vi "采集参数设置.vi"() -> (3 "Cancelled?":bool)   [LabVIEW 2020]
uses:
  global/SettingVariable.vi
  <vilib>/Utility/config.llb/Write Key (Double).vi
  <vilib>/Utility/config.llb/Write Key (Boolean).vi
  <vilib>/Utility/config.llb/Write Key (String).vi
  <vilib>/Utility/config.llb/Write Key (U32).vi
  <vilib>/Utility/config.llb/Write Key (I32).vi
  <vilib>/Utility/config.llb/NI_LVConfig.lvlib
panel:
  in  "电压范围8":cluster{"Numeric":i32, "Numeric":i32}(slide)={"Numeric"=5, "Numeric"=1} scale=-10.0..10.0
  in  "电压范围7":cluster{"Numeric":i32, "Numeric":i32}(slide)={"Numeric"=5, "Numeric"=1} scale=-10.0..10.0
  in  "电压范围6":cluster{"Numeric":i32, "Numeric":i32}(slide)={"Numeric"=5, "Numeric"=1} scale=-10.0..10.0
  in  "电压范围5":cluster{"Numeric":i32, "Numeric":i32}(slide)={"Numeric"=5, "Numeric"=1} scale=-10.0..10.0
  in  "电压范围4":cluster{"Numeric":i32, "Numeric":i32}(slide)={"Numeric"=5, "Numeric"=1} scale=-10.0..10.0
  in  "电压范围3":cluster{"Numeric":i32, "Numeric":i32}(slide)={"Numeric"=5, "Numeric"=1} scale=-10.0..10.0
  in  "电压范围2":cluster{"Numeric":i32, "Numeric":i32}(slide)={"Numeric"=5, "Numeric"=1} scale=-10.0..10.0
  in  "电压范围1":cluster{"Numeric":i32, "Numeric":i32}(slide)={"Numeric"=5, "Numeric"=1} scale=-10.0..10.0
  in  "物理量8下限":sgl format="%#.4g"
  in  "物理量8上限":sgl format="%#.4g"
  in  "物理量7下限":sgl format="%#.4g"
  in  "物理量7上限":sgl format="%#.4g"
  in  "物理量6下限":sgl format="%#.4g"
  in  "物理量6上限":sgl format="%#.4g"
  in  "物理量5下限":sgl format="%#.4g"
  in  "物理量5上限":sgl format="%#.4g"
  in  "物理量4下限":sgl format="%#.4g"
  in  "物理量4上限":sgl format="%#.4g"
  in  "物理量3下限":sgl format="%#.4g"
  in  "物理量3上限":sgl format="%#.4g"
  in  "物理量2下限":sgl format="%#.4g"
  in  "物理量2上限":sgl format="%#.4g"
  in  "物理量1下限":sgl format="%#.4g"
  in  "物理量1上限":sgl format="%#.4g"
  in  "电压标尺8":u16(ring) items=["计数通量LOG", "电压通量", "电流通量LOG", "棒位", "温度", "P2参数", "硼浓度"]
  in  "电压标尺7":u16(ring) items=["计数通量LOG", "电压通量", "电流通量LOG", "棒位", "温度", "P2参数", "硼浓度"]
  in  "电压标尺6":u16(ring) items=["计数通量LOG", "电压通量", "电流通量LOG", "棒位", "温度", "P2参数", "硼浓度"]
  in  "电压标尺5":u16(ring) items=["计数通量LOG", "电压通量", "电流通量LOG", "棒位", "温度", "P2参数", "硼浓度"]
  in  "电压标尺4":u16(ring) items=["计数通量LOG", "电压通量", "电流通量LOG", "棒位", "温度", "P2参数", "硼浓度"]
  in  "电压标尺3":u16(ring) items=["计数通量LOG", "电压通量", "电流通量LOG", "棒位", "温度", "P2参数", "硼浓度"]
  in  "电压标尺2":u16(ring) items=["计数通量LOG", "电压通量", "电流通量LOG", "棒位", "温度", "P2参数", "硼浓度"]
  in  "电压标尺1":u16(ring) items=["计数通量LOG", "电压通量", "电流通量LOG", "棒位", "温度", "P2参数", "硼浓度"]
  in  "电流输入名称2":string
  in  "电流输入名称1":string
  in  "电压输入名称8":string
  in  "电压输入名称7":string
  in  "电压输入名称6":string
  in  "电压输入名称5":string
  in  "电压输入名称4":string
  in  "电压输入名称3":string
  in  "电压输入名称2":string
  in  "电压输入名称1":string
  in  "电流输入2":bool
  in  "电流输入1":bool
  in  "电压输入8":bool
  in  "电压输入7":bool
  in  "电压输入6":bool
  in  "电压输入5":bool
  in  "电压输入4":bool
  in  "电压输入3":bool
  in  "电压输入2":bool
  in  "电压输入1":bool
  in  "取消":bool caption="Cancel Button"
  in  "确定":bool
  in  "采集时间间隔":sgl(knob)=0.5 caption="采集时间间隔(s)：" min=0.5 max=2 step=0.5 scale=0.5..2.0 scale format="%#.1f"
  # "仪器通讯"
  # "电压输入通道"
  # "电流输入通道"
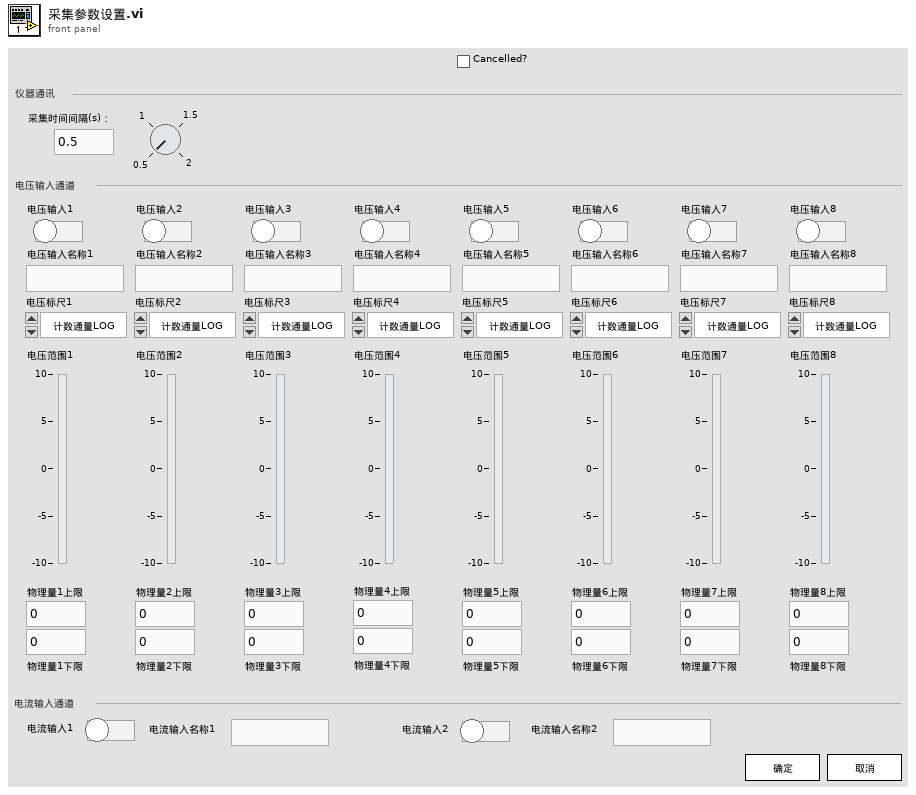
[diagram p1: front panel]
types:
  T1 = cluster{"switch":bool, "name":string, "voltage upper":i32, "voltage lower":i32, "physics upper":dbl, "physics lower":dbl, "scale":u16}[]
  T2 = typedef "NI_LVConfig.lvlib/Config Data RefNum.ctl" = refnum<k1>
  T3 = cluster{"switch":bool, "name":string, "voltage upper":i32, "voltage lower":i32, "physics upper":dbl, "physics lower":dbl, "scale":u16}
  T4 = enum32{"Bad", "Idle", "Run top level", "Running"}
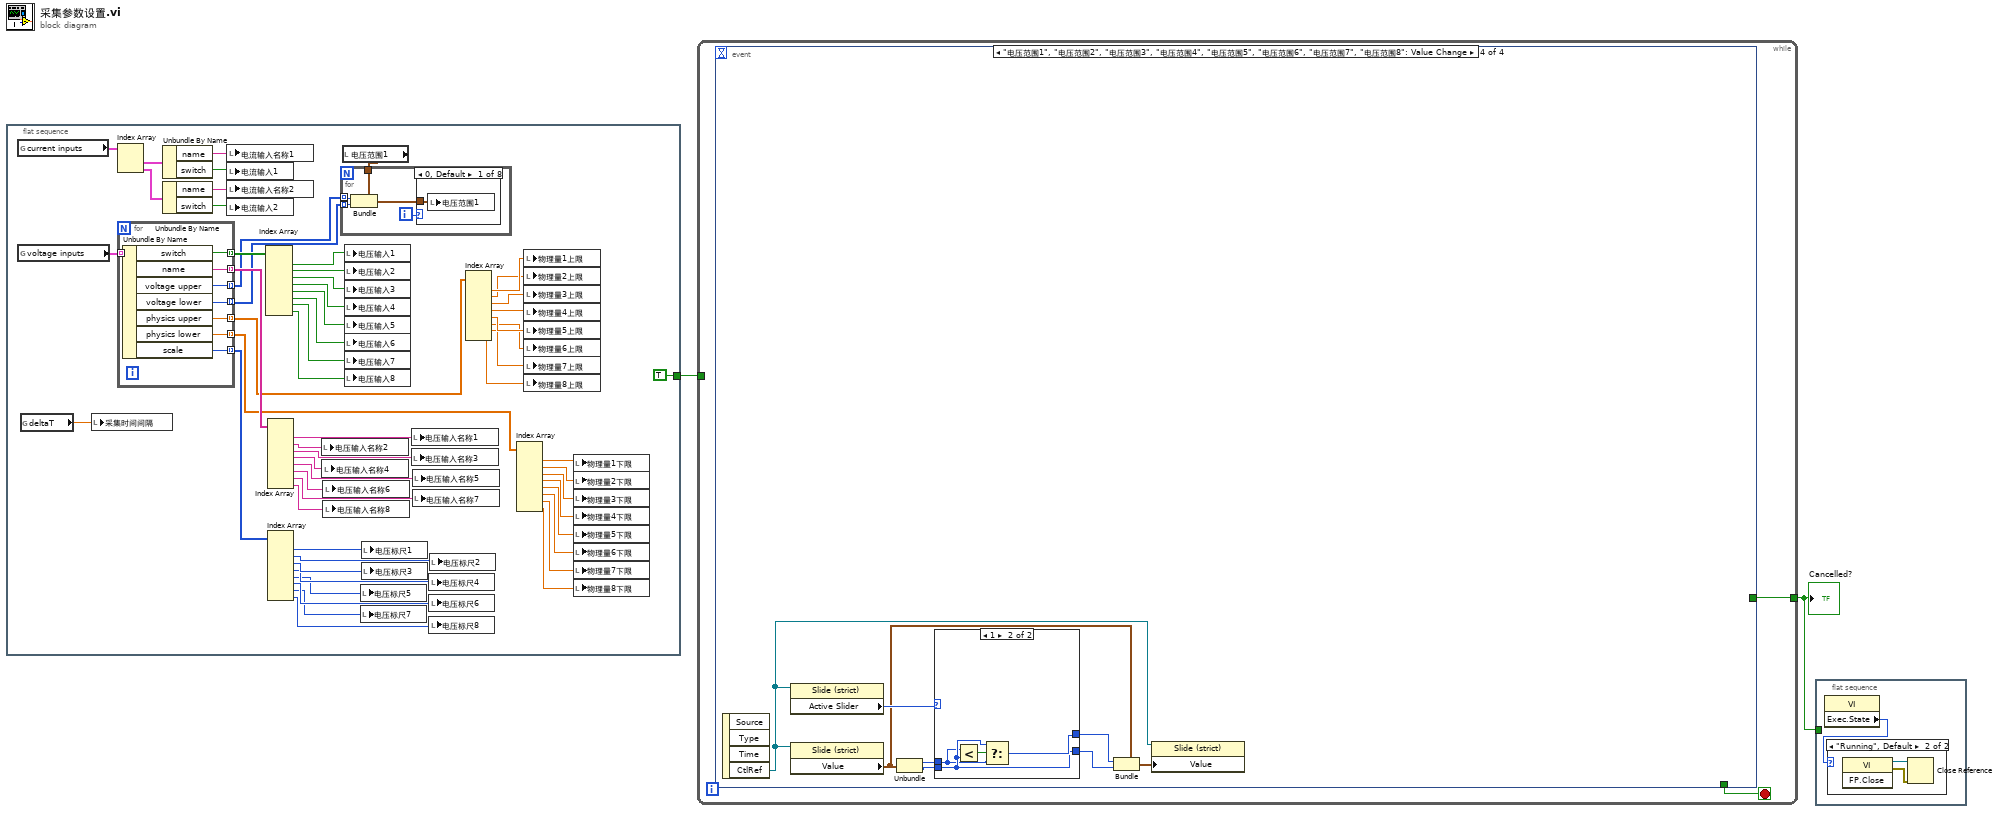
[diagram p0: block diagram]
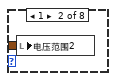
[diagram p3: hidden frame]
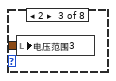
[diagram p4: hidden frame]
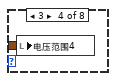
[diagram p5: hidden frame]
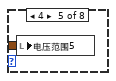
[diagram p6: hidden frame]
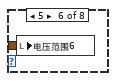
[diagram p7: hidden frame]
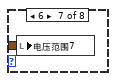
[diagram p8: hidden frame]
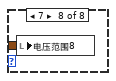
[diagram p9: hidden frame]
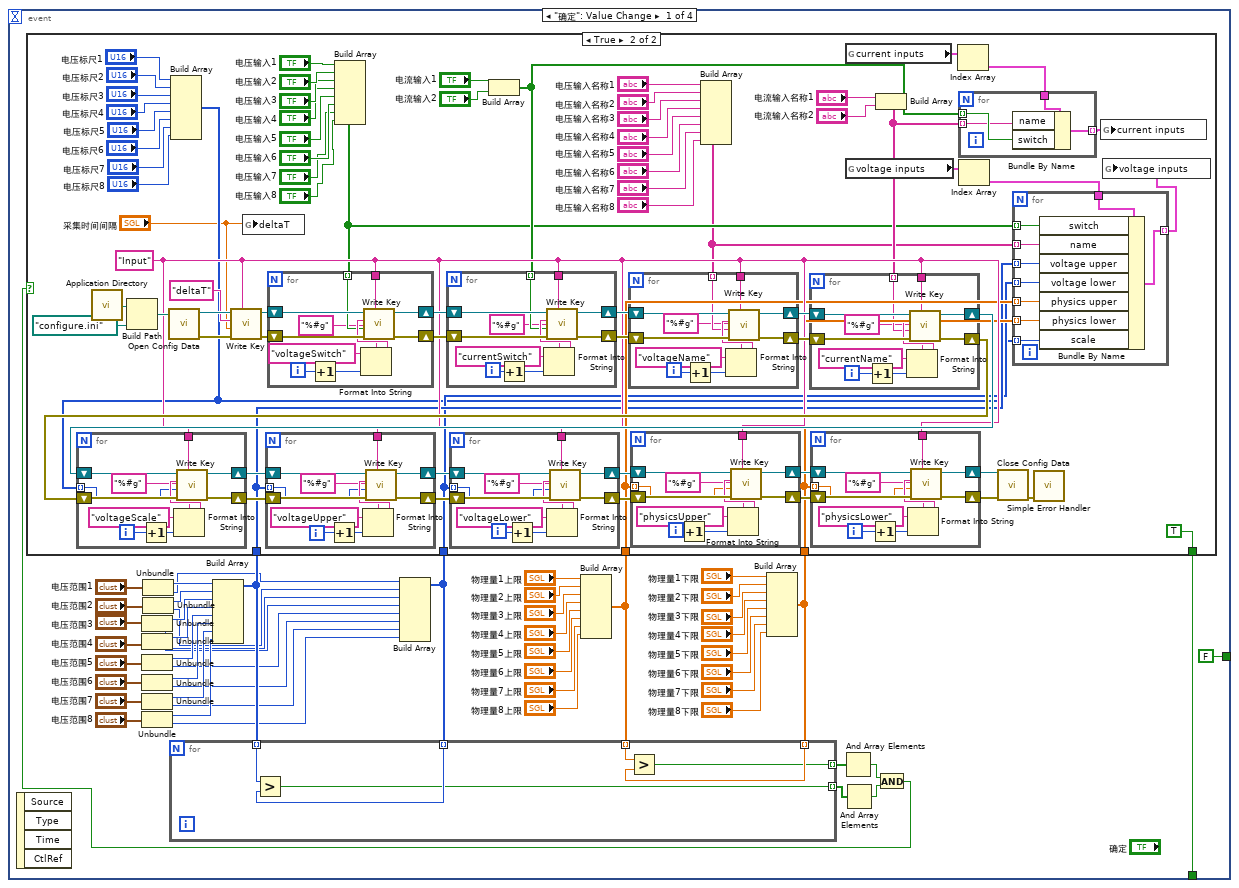
[diagram p10: hidden frame]
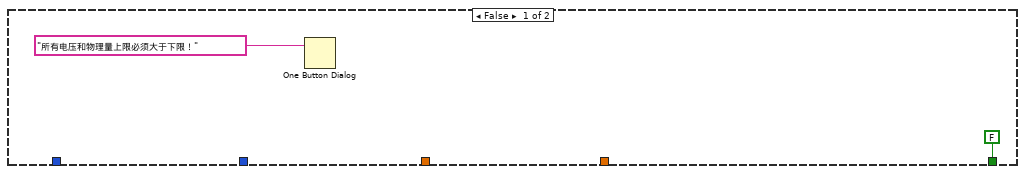
[diagram p11: hidden frame]
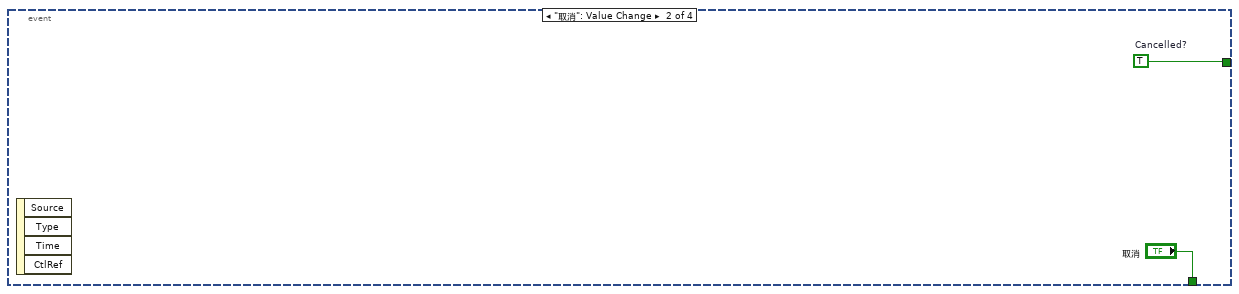
[diagram p12: hidden frame]
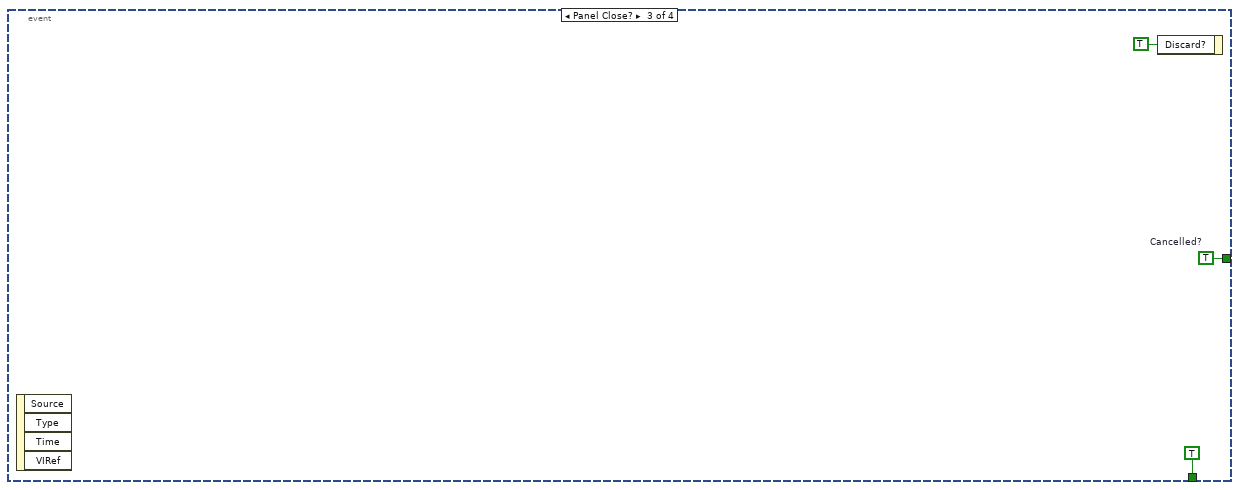
[diagram p13: hidden frame]
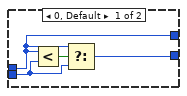
[diagram p14: hidden frame]
diagram:
  n1 = flat-sequence {
    tunnel: [TRUE] -> w2
    frame #0 {
      n2 = global read "SettingVariable.vi" "current inputs"() -> (w59:cluster{"name":string, "switch":bool}[])
      n3 = global read "SettingVariable.vi" "voltage inputs"() -> (w52:T1)
      n4 = global read "SettingVariable.vi" "deltaT"() -> (w60:dbl)
      n5 = local write "采集时间间隔"(w60) -> ()
      n6 = Index Array(array=w59) -> (element #1=w58:cluster{"name":string, "switch":bool}, element #2=w57:cluster{"name":string, "switch":bool})  [unwired: 2 in]
      n7 = for {
        tunnel: w52 -> [w81] mode=indexing
        tunnel: [w80] -> w51 mode=indexing
        tunnel: [w79] -> w41 mode=indexing
        tunnel: [w78] -> w3 mode=indexing
        tunnel: [w77] -> w4 mode=indexing
        tunnel: [w76] -> w23 mode=indexing
        tunnel: [w75] -> w22 mode=indexing
        tunnel: [w74] -> w32 mode=indexing
        n8 = Unbundle By Name(w81) -> ("switch"=w80:bool, "name"=w79:string, "voltage upper"=w78:i32, "voltage lower"=w77:i32, "physics upper"=w76:dbl, "physics lower"=w75:dbl, "scale"=w74:u16)
      }
      n9 = Unbundle By Name(w58) -> ("name"=w56:string, "switch"=w54:bool)
      n10 = Unbundle By Name(w57) -> ("name"=w55:string, "switch"=w53:bool)
      n11 = local write "电流输入名称1"(w56) -> ()
      n12 = local write "电流输入1"(w54) -> ()
      n13 = local write "电流输入名称2"(w55) -> ()
      n14 = local write "电流输入2"(w53) -> ()
      n15 = Index Array(array=w51) -> (element #1=w50:bool, element #2=w49:bool, element #3=w48:bool, element #4=w47:bool, element #5=w46:bool, element #6=w45:bool, element #7=w44:bool, element #8=w43:bool)  [unwired: 8 in]
      n16 = Index Array(array=w41) -> (element #1=w42:string, element #2=w40:string, element #3=w39:string, element #4=w38:string, element #5=w37:string, element #6=w36:string, element #7=w35:string, element #8=w34:string)  [unwired: 8 in]
      n17 = Index Array(array=w32) -> (element #1=w33:u16, element #2=w31:u16, element #3=w30:u16, element #4=w29:u16, element #5=w28:u16, element #6=w27:u16, element #7=w26:u16, element #8=w25:u16)  [unwired: 8 in]
      n18 = local write "电压输入名称2"(w40) -> ()
      n19 = local write "电压输入名称4"(w38) -> ()
      n20 = local write "电压输入名称6"(w36) -> ()
      n21 = local write "电压输入名称8"(w34) -> ()
      n22 = local read "电压范围1"() -> (w5:cluster{"Numeric":i32, "Numeric":i32})
      n23 = for {
        tunnel: w5 -> [w63]
        tunnel: w4 -> [w62] mode=indexing
        tunnel: w3 -> [w61] mode=indexing
        i -> [w64]
        n24 = Bundle(cluster=w63, "Numeric"=w61, "Numeric"=w62) -> (w65:cluster{"Numeric":i32, "Numeric":i32})
        n25 = case shown="0, Default" w64 {
          tunnel: w65 -> [w66 w67 w68 w69 w70 w71 w72 w73]
          frame 0, Default {
            n26 = local write "电压范围1"(w66) -> ()
          }
          frame 1 {
            n27 = local write "电压范围2"(w67) -> ()
          }
          frame 2 {
            n28 = local write "电压范围3"(w68) -> ()
          }
          frame 3 {
            n29 = local write "电压范围4"(w69) -> ()
          }
          frame 4 {
            n30 = local write "电压范围5"(w70) -> ()
          }
          frame 5 {
            n31 = local write "电压范围6"(w71) -> ()
          }
          frame 6 {
            n32 = local write "电压范围7"(w72) -> ()
          }
          frame 7 {
            n33 = local write "电压范围8"(w73) -> ()
          }
        }
      }
      n34 = local write "电压输入1"(w50) -> ()
      n35 = local write "电压输入2"(w49) -> ()
      n36 = local write "电压输入3"(w48) -> ()
      n37 = local write "电压输入4"(w47) -> ()
      n38 = local write "电压输入5"(w46) -> ()
      n39 = local write "电压输入6"(w45) -> ()
      n40 = local write "电压输入7"(w44) -> ()
      n41 = local write "电压输入8"(w43) -> ()
      n42 = local write "电压标尺5"(w28) -> ()
      n43 = local write "电压标尺7"(w26) -> ()
      n44 = local write "电压标尺1"(w33) -> ()
      n45 = local write "电压标尺3"(w30) -> ()
      n46 = local write "电压输入名称1"(w42) -> ()
      n47 = local write "电压输入名称3"(w39) -> ()
      n48 = local write "电压输入名称5"(w37) -> ()
      n49 = local write "电压输入名称7"(w35) -> ()
      n50 = local write "电压标尺4"(w29) -> ()
      n51 = local write "电压标尺6"(w27) -> ()
      n52 = local write "电压标尺8"(w25) -> ()
      n53 = local write "电压标尺2"(w31) -> ()
      n54 = Index Array(array=w23) -> (element #1=w24:dbl, element #2=w21:dbl, element #3=w20:dbl, element #4=w19:dbl, element #5=w18:dbl, element #6=w17:dbl, element #7=w16:dbl, element #8=w15:dbl)  [unwired: 8 in]
      n55 = Index Array(array=w22) -> (element #1=w14:dbl, element #2=w13:dbl, element #3=w12:dbl, element #4=w11:dbl, element #5=w10:dbl, element #6=w9:dbl, element #7=w8:dbl, element #8=w7:dbl)  [unwired: 8 in]
      n56 = local write "物理量1上限"(w24) -> ()
      n57 = local write "物理量2上限"(w21) -> ()
      n58 = local write "物理量3上限"(w20) -> ()
      n59 = local write "物理量4上限"(w19) -> ()
      n60 = local write "物理量5上限"(w18) -> ()
      n61 = local write "物理量6上限"(w17) -> ()
      n62 = local write "物理量7上限"(w16) -> ()
      n63 = local write "物理量8上限"(w15) -> ()
      n64 = local write "物理量1下限"(w14) -> ()
      n65 = local write "物理量2下限"(w13) -> ()
      n66 = local write "物理量3下限"(w12) -> ()
      n67 = local write "物理量4下限"(w11) -> ()
      n68 = local write "物理量5下限"(w10) -> ()
      n69 = local write "物理量6下限"(w9) -> ()
      n70 = local write "物理量7下限"(w8) -> ()
      n71 = local write "物理量8下限"(w7) -> ()
    }
  }
  n72 = while {
    tunnel: w2 -> [_]
    tunnel: [w82] -> w1
    stop <- w83 stop-if-true
    n73 = event shown="[3] \"电压范围1\", \"电压范围2\", \"电压范围3\", \"电压范围4\", \"电压范围5\", \"电压范围6\", \"电压范围7\", \"电压范围8\": Value Change" {
      selector: _ -> [_ _ _ _]
      dyn-events: _ -> [_ _ _ _]
      timeout: _ -> [_ _ _ _]
      tunnel: [w112 "取消" TRUE _] -> w83
      tunnel: [FALSE ("Cancelled?") w328 w330 _] -> w82
      event "确定": Value Change {
        n74 = event-data() -> ()  [unwired: 1 in, 4 out]
        n75 = Unbundle("电压范围3") -> ("Numeric"=w97:i32, "Numeric"=w89:i32)
        n76 = Unbundle("电压范围4") -> ("Numeric"=w96:i32, "Numeric"=w88:i32)
        n77 = Unbundle("电压范围5") -> ("Numeric"=w94:i32, "Numeric"=w87:i32)
        n78 = Unbundle("电压范围6") -> ("Numeric"=w93:i32, "Numeric"=w86:i32)
        n79 = Unbundle("电压范围7") -> ("Numeric"=w92:i32, "Numeric"=w85:i32)
        n80 = Unbundle("电压范围8") -> ("Numeric"=w91:i32, "Numeric"=w84:i32)
        n81 = Unbundle("电压范围1") -> ("Numeric"=w99:i32, "Numeric"=w95:i32)
        n82 = Unbundle("电压范围2") -> ("Numeric"=w98:i32, "Numeric"=w90:i32)
        n83 = Build Array(w99, w98, w97, w96, w94, w93, w92, w91) -> (w121:i32[])
        n84 = Build Array(w95, w90, w89, w88, w87, w86, w85, w84) -> (w120:i32[])
        n85 = Build Array("物理量1上限", "物理量2上限", "物理量3上限", "物理量4上限", "物理量5上限", "物理量6上限", "物理量7上限", "物理量8上限") -> (w119:sgl[])
        n86 = Build Array("物理量1下限", "物理量2下限", "物理量3下限", "物理量4下限", "物理量5下限", "物理量6下限", "物理量7下限", "物理量8下限") -> (w118:sgl[])
        n87 = for {
          tunnel: w121 -> [w327] mode=indexing
          tunnel: w120 -> [w326] mode=indexing
          tunnel: w119 -> [w325] mode=indexing
          tunnel: w118 -> [w324] mode=indexing
          tunnel: [w323] -> w117 mode=indexing
          tunnel: [w322] -> w116 mode=indexing
          n88 = Greater?(x=w327, y=w326) -> (0:w322:bool)
          n89 = Greater?(x=w325, y=w324) -> (0:w323:bool)
        }
        n90 = And Array Elements(Boolean array=w117) -> (logical AND=w114:bool)
        n91 = And Array Elements(Boolean array=w116) -> (logical AND=w115:bool)
        n92 = And(x=w114, y=w115) -> (x .and. y?=w113:bool)
        n93 = case shown="True" w113 {
          tunnel: w121 -> [_ w140]
          tunnel: w120 -> [_ w139]
          tunnel: w119 -> [_ w142]
          tunnel: w118 -> [_ w141]
          tunnel: [FALSE TRUE] -> w112
          frame False {
            n94 = One Button Dialog(message="所有电压和物理量上限必须大于下限！") -> ()  [unwired: 1 in, 1 out]
          }
          frame True {
            w156 = "Input" ("section")
            n95 = call <vilib>:"Application Directory.vi"() -> ("Application Directory"=w180:path)
            n96 = Build Path(base path=w180, name or relative path=path "configure.ini") -> (appended path=w178:path)
            n97 = call <vilib>:"Open Config Data.vi"("configuration file path"=w178) -> ("error out"=w176:errorcluster, "refnum"=w177:T2)  [unwired: 2 in, 7 out]
            n98 = Build Array("电压标尺1", "电压标尺2", "电压标尺3", "电压标尺4", "电压标尺5", "电压标尺6", "电压标尺7", "电压标尺8") -> (w138:u16[])
            n99 = call-poly <vilib>:"Write Key.vi"("section"=w156, "error in (no error)"=w176, "value"="采集时间间隔", "key"="deltaT", "refnum"=w177) -> ("error out"=w173:errorcluster, "refnum out"=w174:T2)  [unwired: 4 in, 1 out]
            n100 = global write "SettingVariable.vi" "deltaT"("采集时间间隔") -> ()
            n101 = Build Array("电压输入1", "电压输入2", "电压输入3", "电压输入4", "电压输入5", "电压输入6", "电压输入7", "电压输入8") -> (w144:bool[])
            n102 = for {
              tunnel: w144 -> [w316] mode=indexing
              shift-right: [w315] -> w172
              shift-left: w174 -> [w321]
              shift-right: [w314] -> w171
              shift-left: w173 -> [w320]
              tunnel: w156 -> [w312]
              i -> [w319]
              n103 = Increment(x=w319) -> (x+1=w311:i32)
              n104 = Format Into String(format string="%#g" ("section"), initial string="voltageSwitch", w311) -> (resulting string=w317:string)  [unwired: 1 in, 1 out]
              n105 = call-poly <vilib>:"Write Key.vi"("section"=w312, "error in (no error)"=w320, "value"=w316, "key"=w317, "refnum"=w321) -> ("error out"=w314:errorcluster, "refnum out"=w315:T2)  [unwired: 4 in, 1 out]
            }
            n106 = Build Array("电流输入1", "电流输入2") -> (w151:bool[])
            n107 = for {
              tunnel: w151 -> [w305] mode=indexing
              shift-right: [w303] -> w169
              shift-left: w172 -> [w310]
              shift-right: [w304] -> w170
              shift-left: w171 -> [w309]
              tunnel: w156 -> [w301]
              i -> [w308]
              n108 = Increment(x=w308) -> (x+1=w300:i32)
              n109 = Format Into String(format string="%#g" ("section"), initial string="currentSwitch", w300) -> (resulting string=w306:string)  [unwired: 1 in, 1 out]
              n110 = call-poly <vilib>:"Write Key.vi"("section"=w301, "error in (no error)"=w309, "value"=w305, "key"=w306, "refnum"=w310) -> ("error out"=w304:errorcluster, "refnum out"=w303:T2)  [unwired: 4 in, 1 out]
            }
            n111 = Build Array("电压输入名称1", "电压输入名称2", "电压输入名称3", "电压输入名称4", "电压输入名称5", "电压输入名称6", "电压输入名称7", "电压输入名称8") -> (w143:string[])
            n112 = for {
              tunnel: w143 -> [w294] mode=indexing
              tunnel: w156 -> [w292]
              shift-right: [w291] -> w168
              shift-left: w169 -> [w299]
              shift-right: [w290] -> w167
              shift-left: w170 -> [w298]
              i -> [w297]
              n113 = Increment(x=w297) -> (x+1=w289:i32)
              n114 = Format Into String(format string="%#g" ("section"), initial string="voltageName", w289) -> (resulting string=w295:string)  [unwired: 1 in, 1 out]
              n115 = call-poly <vilib>:"Write Key.vi"("section"=w292, "error in (no error)"=w298, "value"=w294, "key"=w295, "refnum"=w299) -> ("error out"=w290:errorcluster, "refnum out"=w291:T2)  [unwired: 4 in, 1 out]
            }
            n116 = global read "SettingVariable.vi" "current inputs"() -> (w150:cluster{"name":string, "switch":bool}[])
            n117 = global read "SettingVariable.vi" "voltage inputs"() -> (w147:T1)
            n118 = Build Array("电流输入名称1", "电流输入名称2") -> (w152:string[])
            n119 = for {
              tunnel: w152 -> [w283] mode=indexing
              tunnel: w156 -> [w281]
              shift-right: [w280] -> w158
              shift-left: w168 -> [w288]
              shift-right: [w279] -> w157
              shift-left: w167 -> [w287]
              i -> [w286]
              n120 = Increment(x=w286) -> (x+1=w278:i32)
              n121 = Format Into String(format string="%#g" ("section"), initial string="currentName", w278) -> (resulting string=w284:string)  [unwired: 1 in, 1 out]
              n122 = call-poly <vilib>:"Write Key.vi"("section"=w281, "error in (no error)"=w287, "value"=w283, "key"=w284, "refnum"=w288) -> ("error out"=w279:errorcluster, "refnum out"=w280:T2)  [unwired: 4 in, 1 out]
            }
            n123 = for {
              tunnel: w156 -> [w228]
              shift-right: [w227] -> w160
              shift-left: w158 -> [w233]
              shift-right: [w226] -> w159
              shift-left: w157 -> [w232]
              tunnel: w138 -> [w225] mode=indexing
              i -> [w224]
              n124 = Increment(x=w224) -> (x+1=w223:i32)
              n125 = Format Into String(format string="%#g" ("section"), initial string="voltageScale", w223) -> (resulting string=w230:string)  [unwired: 1 in, 1 out]
              n126 = call-poly <vilib>:"Write Key.vi"("section"=w228, "error in (no error)"=w232, "value"=w225, "key"=w230, "refnum"=w233) -> ("error out"=w226:errorcluster, "refnum out"=w227:T2)  [unwired: 4 in, 1 out]
            }
            n127 = for {
              tunnel: w156 -> [w271]
              shift-right: [w270] -> w166
              shift-left: w160 -> [w277]
              shift-right: [w269] -> w165
              shift-left: w159 -> [w276]
              tunnel: w140 -> [w268] mode=indexing
              i -> [w275]
              n128 = Increment(x=w275) -> (x+1=w267:i32)
              n129 = Format Into String(format string="%#g" ("section"), initial string="voltageUpper", w267) -> (resulting string=w273:string)  [unwired: 1 in, 1 out]
              n130 = call-poly <vilib>:"Write Key.vi"("section"=w271, "error in (no error)"=w276, "value"=w268, "key"=w273, "refnum"=w277) -> ("error out"=w269:errorcluster, "refnum out"=w270:T2)  [unwired: 4 in, 1 out]
            }
            n131 = for {
              tunnel: w156 -> [w260]
              shift-right: [w259] -> w164
              shift-left: w166 -> [w266]
              shift-right: [w258] -> w163
              shift-left: w165 -> [w265]
              tunnel: w139 -> [w257] mode=indexing
              i -> [w264]
              n132 = Increment(x=w264) -> (x+1=w256:i32)
              n133 = Format Into String(format string="%#g" ("section"), initial string="voltageLower", w256) -> (resulting string=w262:string)  [unwired: 1 in, 1 out]
              n134 = call-poly <vilib>:"Write Key.vi"("section"=w260, "error in (no error)"=w265, "value"=w257, "key"=w262, "refnum"=w266) -> ("error out"=w258:errorcluster, "refnum out"=w259:T2)  [unwired: 4 in, 1 out]
            }
            n135 = for {
              tunnel: w156 -> [w249]
              shift-right: [w248] -> w162
              shift-left: w164 -> [w255]
              shift-right: [w247] -> w161
              shift-left: w163 -> [w254]
              tunnel: w142 -> [w246] mode=indexing
              i -> [w253]
              n136 = Increment(x=w253) -> (x+1=w245:i32)
              n137 = Format Into String(format string="%#g" ("section"), initial string="physicsUpper", w245) -> (resulting string=w251:string)  [unwired: 1 in, 1 out]
              n138 = call-poly <vilib>:"Write Key.vi"("section"=w249, "error in (no error)"=w254, "value"=w246, "key"=w251, "refnum"=w255) -> ("error out"=w247:errorcluster, "refnum out"=w248:T2)  [unwired: 4 in, 1 out]
            }
            n139 = for {
              tunnel: w156 -> [w238]
              shift-right: [w237] -> w154
              shift-left: w162 -> [w244]
              shift-right: [w236] -> w155
              shift-left: w161 -> [w243]
              tunnel: w141 -> [w235] mode=indexing
              i -> [w242]
              n140 = Increment(x=w242) -> (x+1=w234:i32)
              n141 = Format Into String(format string="%#g" ("section"), initial string="physicsLower", w234) -> (resulting string=w240:string)  [unwired: 1 in, 1 out]
              n142 = call-poly <vilib>:"Write Key.vi"("section"=w238, "error in (no error)"=w243, "value"=w235, "key"=w240, "refnum"=w244) -> ("error out"=w236:errorcluster, "refnum out"=w237:T2)  [unwired: 4 in, 1 out]
            }
            n143 = Index Array(array=w150) -> (element=w149:cluster{"name":string, "switch":bool})  [unwired: 1 in]
            n144 = for {
              tunnel: w152 -> [w220] mode=indexing
              tunnel: w151 -> [w221] mode=indexing
              tunnel: w149 -> [w222]
              tunnel: [w219] -> w148 mode=indexing
              n145 = Bundle By Name(cluster=w222, "name"=w220, "switch"=w221) -> (w219:cluster{"name":string, "switch":bool})
            }
            n146 = Index Array(array=w147) -> (element=w146:T3)  [unwired: 1 in]
            n147 = call <vilib>:"Close Config Data.vi"("error in (no error)"=w155, "refnum"=w154) -> ("error out"=w181:errorcluster)  [unwired: 1 in, 8 out]
            n148 = for {
              tunnel: w146 -> [w218]
              tunnel: [w217] -> w145 mode=indexing
              tunnel: w144 -> [w216] mode=indexing
              tunnel: w143 -> [w215] mode=indexing
              tunnel: w142 -> [w214] mode=indexing
              tunnel: w141 -> [w213] mode=indexing
              tunnel: w140 -> [w212] mode=indexing
              tunnel: w139 -> [w211] mode=indexing
              tunnel: w138 -> [w210] mode=indexing
              n149 = Bundle By Name(cluster=w218, "switch"=w216, "name"=w215, "voltage upper"=w212, "voltage lower"=w211, "physics upper"=w214, "physics lower"=w213, "scale"=w210) -> (w217:T3)
            }
            n150 = call <vilib>:"Simple Error Handler.vi"("error in (no error)"=w181) -> ()  [unwired: 1 in, 8 out]
            n151 = global write "SettingVariable.vi" "current inputs"(w148) -> ()
            n152 = global write "SettingVariable.vi" "voltage inputs"(w145) -> ()
          }
        }
      }
      event "取消": Value Change {
        w328 = TRUE  # Cancelled?
        n153 = event-data() -> ()  [unwired: 1 in, 4 out]
      }
      event Panel Close? {
        w330 = TRUE  # Cancelled?
        n154 = event-data() -> ()  [unwired: 1 in, 4 out]
        n155 = event-data("Discard?"=TRUE) -> ()  [unwired: 1 in, 1 out]
      }
      event "电压范围1", "电压范围2", "电压范围3", "电压范围4", "电压范围5", "电压范围6", "电压范围7", "电压范围8": Value Change {
        n156 = event-data() -> ("CtlRef"=w333:refnum<vi>)  [unwired: 1 in, 3 out]
        n157 = property class="Slide (strict)"(reference=w333) -> ("Active Slider"=w340:i32)  [unwired: 1 in, 2 out]
        n158 = property class="Slide (strict)"(reference=w333) -> ("Value"=w336:cluster{"Numeric":i32, "Numeric":i32})  [unwired: 1 in, 2 out]
        n159 = Unbundle(w336) -> ("Numeric"=w339:i32, "Numeric"=w338:i32)
        n160 = case shown="1" w340 {
          tunnel: w339 -> [w341 w345]
          tunnel: w338 -> [w343 w346]
          tunnel: [w342 w346] -> w335
          tunnel: [w341 w347] -> w334
          frame 0, Default {
            n161 = Less?(x=w341, y=w343) -> (x < y?=w344:bool)
            n162 = Select(t=w341, s=w344, f=w343) -> (s? t:f=w342:i32)
          }
          frame 1 {
            n163 = Less?(x=w345, y=w346) -> (x < y?=w348:bool)
            n164 = Select(t=w346, s=w348, f=w345) -> (s? t:f=w347:i32)
          }
        }
        n165 = Bundle(cluster=w336, "Numeric"=w334, "Numeric"=w335) -> (w337:cluster{"Numeric":i32, "Numeric":i32})
        n166 = property class="Slide (strict)"(reference=w333, "Value"=w337) -> ()  [unwired: 1 in, 2 out]
      }
    }
  }
  "Cancelled?" <- w1
  n167 = flat-sequence {
    tunnel: w1 -> [_]
    frame #0 {
      n168 = property class="VI"() -> ("Exec.State"=w349:T4)  [unwired: 2 in, 2 out]
      n169 = case shown="\"Running\", Default" w349 {
        frame "Run top level" {
        }
        frame "Running", Default {
          n170 = invoke class="VI" method="FP.Close"() -> (reference out=w350:refnum<vi>, error out=w351:errorcluster)  [unwired: 3 in, 1 out]
          n171 = Close Reference(reference=w350, error in (no error)=w351) -> ()  [unwired: 1 out]
        }
      }
    }
  }
